vi "Test State Machine API.vi"() -> (0 "error out":errorcluster)   [LabVIEW 2019, in "LVCOOOP Tests.lvlib" / "State Machine API.lvlib"]
uses:
  State Machine API.lvlib
  types/Action.ctl
  types/Guard.ctl
  types/State.ctl
  types/Data.ctl
  types/Event.ctl
  fe5d10cc-a1bd-4d71-b2bc-3438492534bb.vi
  ac5a1e06-9b32-4d4e-8582-5c5f0ab05c8d.vi
  fe5d10cc-a1bd-4d71-b2bc-3438492534bb.vi/f5fe9a64-4f5f-4549-8de0-991e74ccd67d.vi
  fe5d10cc-a1bd-4d71-b2bc-3438492534bb.vi/79bdfb0b-b517-4db2-b6a9-48ebe70fa18d.vi
  fe5d10cc-a1bd-4d71-b2bc-3438492534bb.vi/693ad457-2bef-47f4-a8f5-416a628c2cc4.vi
  fe5d10cc-a1bd-4d71-b2bc-3438492534bb.vi/14c2fa41-2690-4afc-a7ad-1d0092f437bc.vi
  fe5d10cc-a1bd-4d71-b2bc-3438492534bb.vi/12487ba8-958f-4fe1-be9b-13051b60aeae.vi
  fe5d10cc-a1bd-4d71-b2bc-3438492534bb.vi/9cb8b2c5-5086-43b3-bada-c85ff5d305c6.vi
  fe5d10cc-a1bd-4d71-b2bc-3438492534bb.vi/b9bf764c-b2fb-4daf-9d1a-1922b37ccbff.vi
  fe5d10cc-a1bd-4d71-b2bc-3438492534bb.vi/014d1cbe-8d42-4a46-93c4-322b08c8909a.vi
  fe5d10cc-a1bd-4d71-b2bc-3438492534bb.vi/682f75b5-eedf-4d6b-8010-28d6c04d8a8d.vi
  fe5d10cc-a1bd-4d71-b2bc-3438492534bb.vi/868c6fc5-9f0d-48cc-825a-735a748dcbcc.vi
  LVCOOOP/State Machine API/subVIs/strip_string.vi
  fe5d10cc-a1bd-4d71-b2bc-3438492534bb.vi/20baebe6-7278-42c3-9d57-ca261d5426dc.vi
  fe5d10cc-a1bd-4d71-b2bc-3438492534bb.vi/94c5739b-341e-434b-8158-f3dff53852ac.vi
  fe5d10cc-a1bd-4d71-b2bc-3438492534bb.vi/3638fad2-a325-4f19-9c40-b9dd23aa2e66.vi
  fe5d10cc-a1bd-4d71-b2bc-3438492534bb.vi/5efa6e29-2cca-4190-b175-986021e14611.vi
  fe5d10cc-a1bd-4d71-b2bc-3438492534bb.vi/53cf1996-0833-4fca-b5a7-e66e6034bec3.vi
  fe5d10cc-a1bd-4d71-b2bc-3438492534bb.vi/d79b0c1a-d9e2-420b-82d9-d87e56d2323c.vi
  <vilib>/Utility/error.llb/Trim Whitespace.vi
  Test Guards.vi
  Test Actions.vi
panel:
  out "pass?":bool
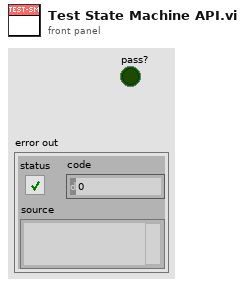
[diagram p1: front panel]
types:
  T1 = typedef "LVCOOOP Tests.lvlib/State Machine API.lvlib/State.ctl" = enum16{"state1", "state2", "state3", "state4"}
  T2 = typedef "LVCOOOP Tests.lvlib/State Machine API.lvlib/Event.ctl" = enum16{"event1", "event2"}
  T3 = typedef "LVCOOOP Tests.lvlib/State Machine API.lvlib/Data.ctl" = cluster{"test value":bool}
  T4 = typedef "LVCOOOP Tests.lvlib/State Machine API.lvlib/Guard.ctl" = enum16{"guard1"}
  T5 = typedef "LVCOOOP Tests.lvlib/State Machine API.lvlib/Action.ctl" = enum16{"action1"}
  T6 = map{T1, map{T2, cluster{"State Type":T1, "Action Type":T5, bool, "Guard Type":T4, bool}[]}}
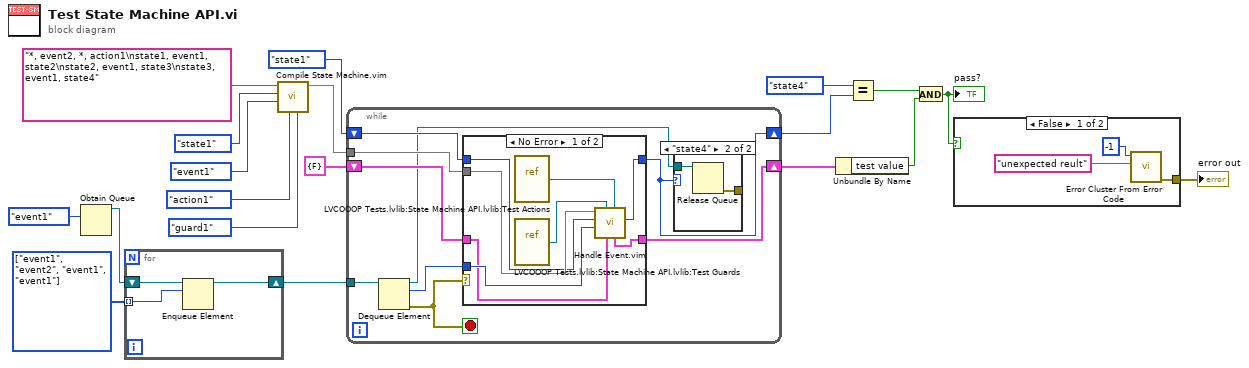
[diagram p0: block diagram]
diagram:
  w8 = T2[] [enum."event1", enum."event2", enum."event1", enum."event1"] items=["event1", "event2"]
  n1 = Obtain Queue(element data type=Event."event1" ("Event")) -> (queue out=w14:refnum<queue>)  [unwired: 4 in, 2 out]
  n2 = for {
    shift-right: [w21] -> w9
    shift-left: w14 -> [w22]
    tunnel: w8 -> [w20] mode=indexing
    n3 = Enqueue Element(queue=w22, element=w20) -> (queue out=w21:refnum<queue>)  [unwired: 2 in, 2 out]
  }
  n4 = call "Compile State Machine.vim"("Guard Type"=Guard."guard1" ("Guard"), "Action Type"=Action."action1" ("Action"), "Event Type"=Event."event1" ("Event"), "State Type"=State."state1" ("State"), "state machine definition"="*, event2, *, action1\nstate1, event1, state2\nstate2, event1, state3\nstate3, event1, state4") -> ("map"=w18:T6)  [unwired: 5 in, 1 out]
  n5 = while {
    tunnel: w18 -> [w29]
    shift-right: [w23] -> w7
    shift-left: State."state1" ("State") -> [w28]
    shift-right: [w31] -> w5
    shift-left: T3 {"test value"=FALSE} ("Data") -> [w26]
    tunnel: w9 -> [w30]
    stop <- w25 stop-if-true
    n6 = Dequeue Element(queue=w30) -> (queue out=w24:refnum<queue>, element=w27:T2, error out=w25:errorcluster)  [unwired: 2 in, 1 out]
    n7 = case shown="No Error" w25 {
      tunnel: [w41 w43] -> w31
      tunnel: [w40 w42] -> w23
      tunnel: w29 -> [w39 _]
      tunnel: w28 -> [w38 w42]
      tunnel: w27 -> [w37 _]
      tunnel: w26 -> [w36 w43]
      frame No Error {
        n8 = vi-ref "LVCOOOP Tests.lvlib:State Machine API.lvlib:Test Actions.vi"() -> (w34:refnum<vi>)
        n9 = vi-ref "LVCOOOP Tests.lvlib:State Machine API.lvlib:Test Guards.vi"() -> (w35:refnum<vi>)
        n10 = call "Handle Event.vim"("actions"=w34, "state data in"=w36, "guards"=w35, "event"=w37, "state in"=w38, "map"=w39) -> ("state out"=w40:T1, "state data out"=w41:T3)  [unwired: 2 in, 2 out]
      }
      frame Error {
      }
    }
    n11 = case shown="\"state4\"" w23 {
      tunnel: w24 -> [_ w33]
      tunnel: [_ w32] -> _
      frame Default {
      }
      frame "state4" {
        n12 = Release Queue(queue=w33) -> (error out=w32:errorcluster)  [unwired: 2 in, 2 out]
      }
    }
  }
  n13 = Unbundle By Name(w5) -> ("test value"=w3:bool)
  n14 = Equal?(x=State."state4", y=w7) -> (x = y?=w4:bool)
  n15 = And(x=w4, y=w3) -> (x .and. y?=w2:bool)
  "pass?" <- w2
  n16 = case shown="False" w2 {
    tunnel: [w44 _] -> w1
    frame False {
      n17 = call <vilib>:"Error Cluster From Error Code.vi"("error message (\"\")"="unexpected reult" ("error message (\"\")"), "error code (0)"=-1) -> ("error out"=w44:errorcluster)  [unwired: 7 in]
    }
    frame True {
    }
  }
  "error out" <- w1
